vi "RVC Quaternion Transformation.vi"() -> ()   [LabVIEW 2013]
uses:
  <vilib>/Analysis/Matrix/Datatypes/RealMatrix.ctl
  <vilib>/robotics/Kinematics/Quaternion.ctl
  <vilib>/robotics/Kinematics/Divide Quaternion by Quaternion.vi
  <vilib>/robotics/Kinematics/Inverse Quaternion.vi
  <vilib>/robotics/Kinematics/RotateX.vi
  <vilib>/robotics/Kinematics/RotateY.vi
  <vilib>/robotics/Kinematics/RotateZ.vi
  <vilib>/Analysis/baseanly.llb/A x B.vi
  <vilib>/Analysis/baseanly.llb/Real A x B.vi
  <vilib>/Analysis/baseanly.llb/Outer Product.vi
  <vilib>/Analysis/baseanly.llb/Real Outer Product.vi
  <vilib>/robotics/Kinematics/Create Lie Group Matrix.vi
  <vilib>/Analysis/_algsub.llb/Vector Norm.vi
  <vilib>/Analysis/_algsub.llb/Real Vector Norm.vi
  <vilib>/Analysis/baseanly.llb/Dot Product.vi
  <vilib>/Analysis/baseanly.llb/Real Dot Product.vi
  <vilib>/robotics/Kinematics/Multiply Quaternion by Quaternion.vi
  <vilib>/robotics/Kinematics/Rotation Matrix to Angle Vector.vi
  <vilib>/Analysis/Matrix/Numeric/Multiply/Multiply.vi
  <vilib>/Analysis/Matrix/Numeric/Multiply/Multiply - RM,R.vi
  <vilib>/Analysis/Matrix/Numeric/Multiply/Multiply - R,RM.vi
  <vilib>/Analysis/Matrix/Numeric/Add/Add.vi
  <vilib>/Analysis/Matrix/Numeric/Add/Add - RM,RM.vi
  <vilib>/robotics/Kinematics/NI_Kinematics.lvlib
  <vilib>/Analysis/Matrix/NI_Matrix.lvlib
panel:
  out "rotated vector":dbl[](array[numeric])
  out "rotation matrix":T1
  out "3D Picture":refnum<vi>(3d-picture)
  out "q / q~":dbl[](array[numeric])=[1.0, 1.0, 1.0] format="%#_4g"
  out "q * q~":dbl[](array[numeric])=[1.0, 1.0, 1.0] format="%#_4g"
  out "Conjugate (q~)":dbl[](array[numeric])=[1.0, 1.0, 1.0]
  out "normalized quaternion":dbl
  out "Position (q)":dbl[](array[numeric])=[1.0, 1.0, 1.0]
  out "transformation matrix":picture
  in  "Position":dbl[](array[numeric])=[1.0, 1.0, 1.0]
  in  "angles":cluster{"roll":dbl, "pitch":dbl, "yaw":dbl}={"roll"=0.1, "pitch"=0.2, "yaw"=0.3} {"roll" scale=-3.14..3.14; "pitch" scale=-3.14..3.14; "yaw" scale=-1.54..1.54}
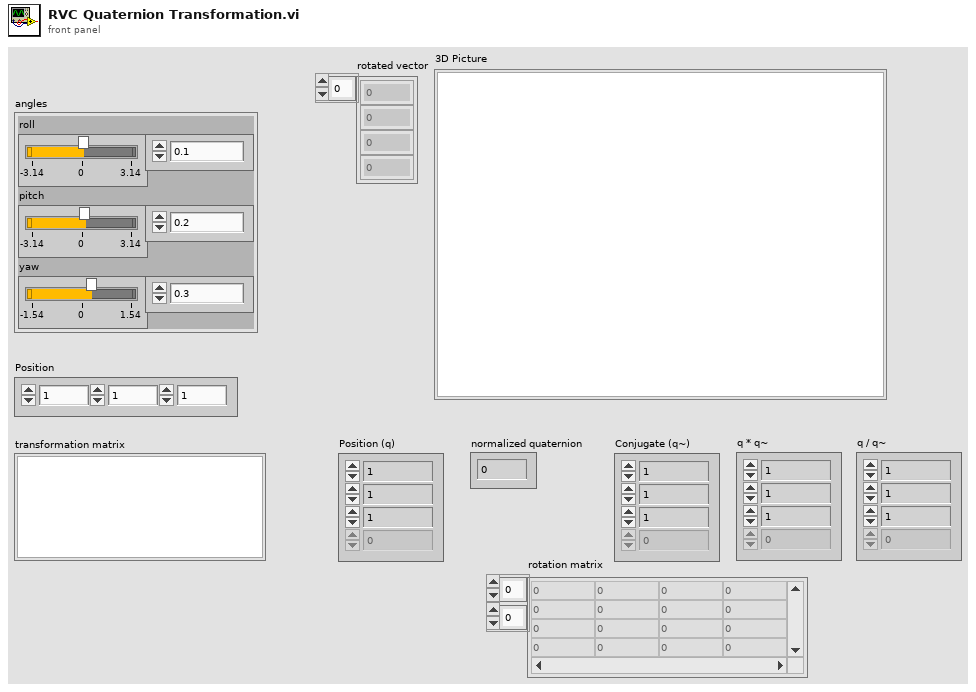
[diagram p1: front panel]
types:
  T1 = typedef "NI_Matrix.lvlib/RealMatrix.ctl" = dbl[][]
  T2 = typedef "NI_Kinematics.lvlib/Quaternion.ctl" = dbl[]
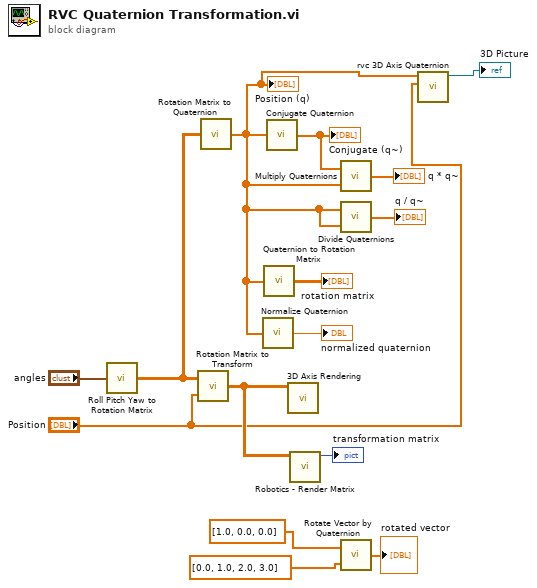
[diagram p0: block diagram]
diagram:
  n1 = call <vilib>:"Roll Pitch Yaw to Rotation Matrix.vi"("angles"="angles") -> ("rotation matrix"=w11:T1)
  n2 = call <vilib>:"Rotation Matrix to Transform.vi"("translation vector"="Position", "rotation matrix"=w11) -> ("transform"=w10:T1)
  n3 = call <vilib>:"Rotation Matrix to Quaternion.vi"("rotation matrix"=w11) -> ("quaternion"=w3:T2)
  "Position (q)" <- w3
  n4 = call <vilib>:"Normalize Quaternion.vi"("quaternion"=w3) -> ("normalized quaternion"=→"normalized quaternion":dbl)
  n5 = call <vilib>:"Quaternion to Rotation Matrix.vi"("quaternion"=w3) -> ("rotation matrix"=→"rotation matrix":T1)
  n6 = call <vilib>:"Conjugate Quaternion.vi"("quaternion"=w3) -> ("conjugate"=w8:T2)
  "Conjugate (q~)" <- w8
  n7 = call "3D Axis Rendering.vi"("rotation matrix"=w10) -> ()  [unwired: 9 in, 2 out]
  n8 = call "Robotics - Render Matrix.vi"("A"=w10) -> ("picture out"=→"transformation matrix":picture)  [unwired: 10 in]
  n9 = call-poly <vilib>:"Multiply Quaternions.vi"("y"=w3, "quaternion"=w8) -> ("product"=→"q * q~":T2)
  n10 = call-poly <vilib>:"Divide Quaternions.vi"("y"=w3, "quaternion"=w3) -> ("quotient"=→"q / q~":T2)
  n11 = call <vilib>:"Rotate Vector by Quaternion.vi"("quaternion"=T2 [0.0, 1.0, 2.0, 3.0], "vector"=dbl[] [1.0, 0.0, 0.0]) -> ("rotated vector"=→"rotated vector":dbl[])  [unwired: 1 in]
  n12 = call "rvc 3D Axis Quaternion.vi"("translation vector"="Position", "quaternion"=w3) -> ("SceneNode out"=→"3D Picture":refnum<vi>)  [unwired: 9 in]
